vi "Read TCP FIFO MTi.vi"(6 "Error In":errorcluster, 9 "Vessel.lvclass":refnum<class "Vessel.lvclass">) -> (0 "Error Out":errorcluster, 3 "Vessel.lvclass 2":refnum<class "Vessel.lvclass">)   [LabVIEW 2014, in "Vessel.lvclass"]
uses:
  Vessel.lvclass
panel:
  out "MT_DATA":sgl[](array[numeric])
  out "MT_BITS":u8[](array[numeric])
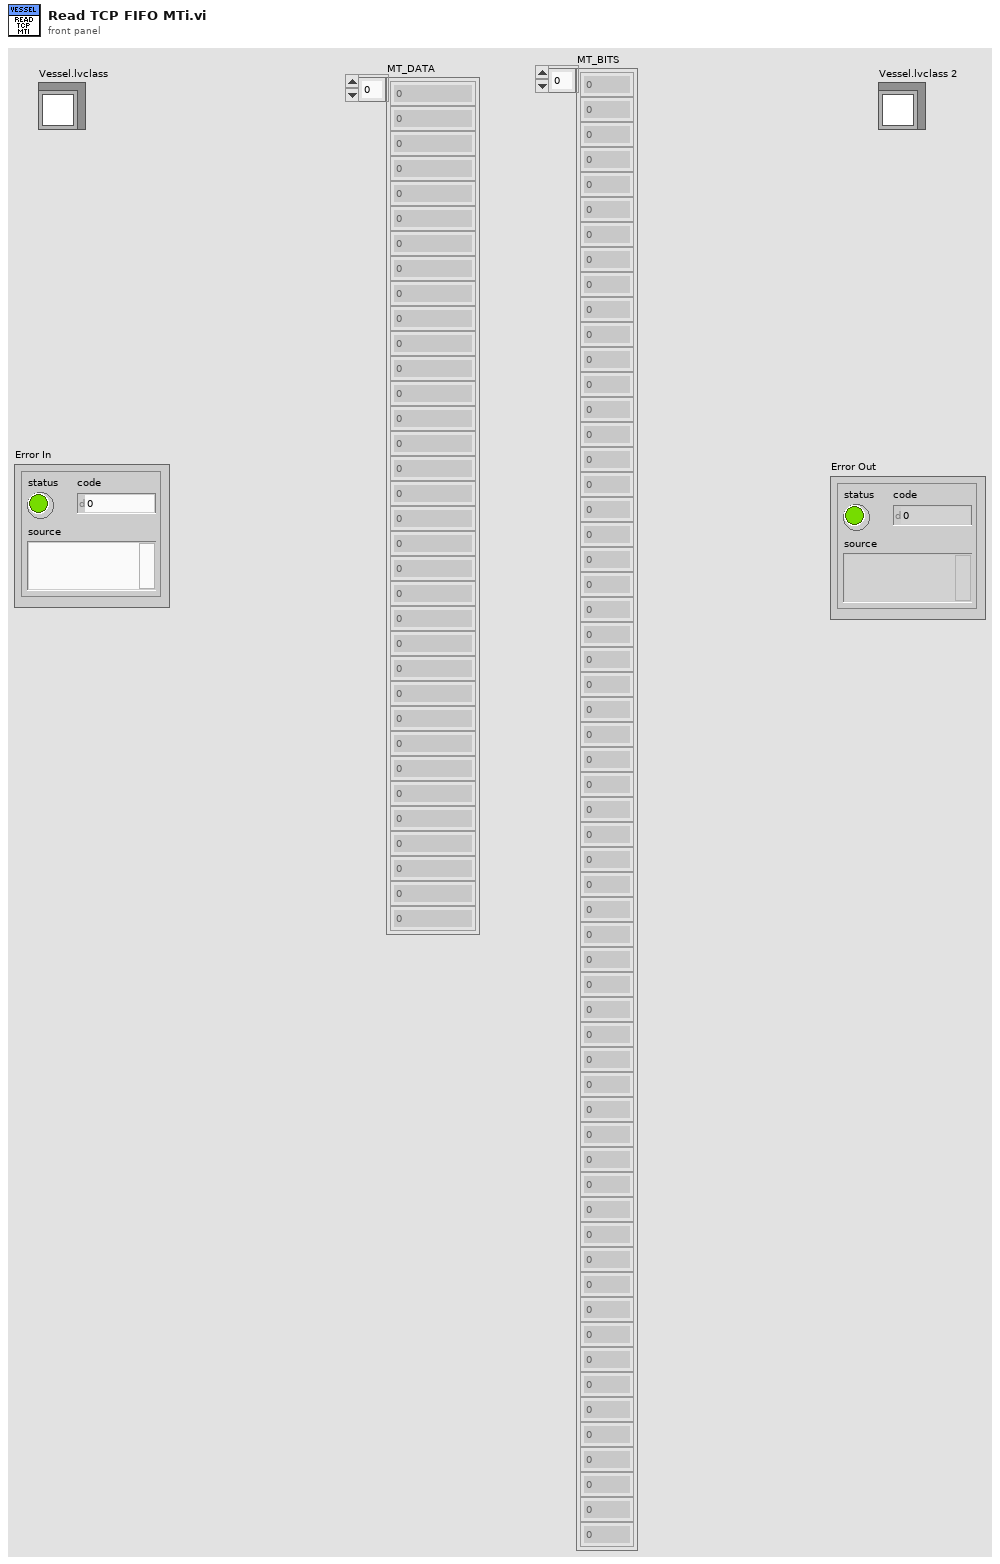
[diagram p1: front panel]
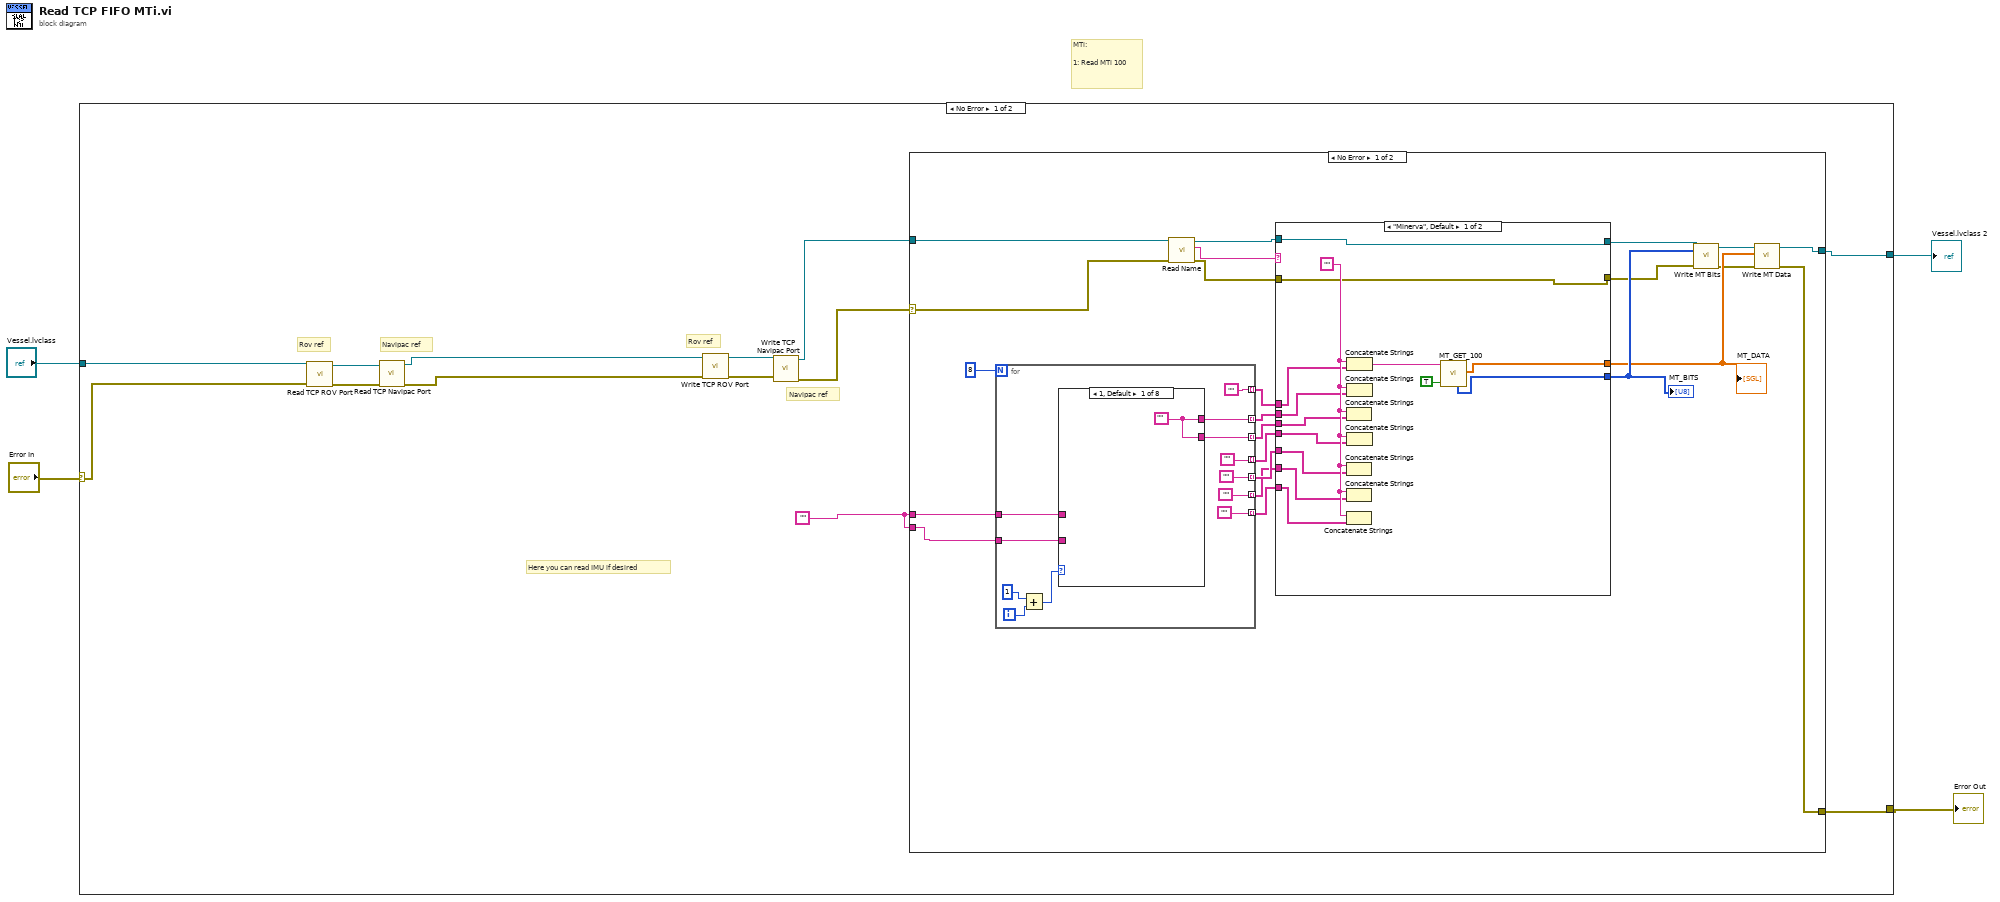
[diagram p0: block diagram]
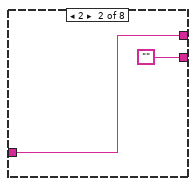
[diagram p2: hidden frame]
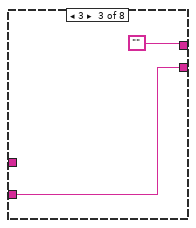
[diagram p3: hidden frame]
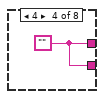
[diagram p4: hidden frame]
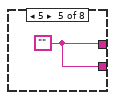
[diagram p5: hidden frame]
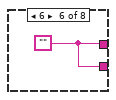
[diagram p6: hidden frame]
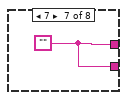
[diagram p7: hidden frame]
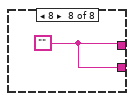
[diagram p8: hidden frame]
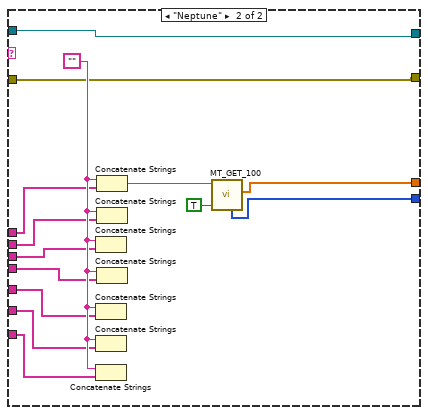
[diagram p9: hidden frame]
diagram:
  # "MTi:\n\n1: Read MTi 100"
  n1 = case shown="No Error" "Error In" {
    selector: "Error In" -> [w15 w93]
    tunnel: "Vessel.lvclass" -> [w14 w94]
    tunnel: [w17 w93] -> w2
    tunnel: [w16 w94] -> w1
    frame No Error {
      w5 = ""
      # "Here you can read IMU if desired"
      # "Navipac ref"
      # "Rov ref"
      # "Navipac ref"
      # "Rov ref"
      n2 = call-dynamic "Read TCP ROV Port.vi"("error in (no error)"=w15, "Vessel in"=w14) -> ("error out"=w12:errorcluster, "Vessel out"=w13:refnum<class "Vessel.lvclass">)  [unwired: 7 in, 1 out]
      n3 = call-dynamic "Read TCP Navipac Port.vi"("error in (no error)"=w12, "Vessel in"=w13) -> ("error out"=w6:errorcluster, "Vessel out"=w9:refnum<class "Vessel.lvclass">)  [unwired: 7 in, 1 out]
      n4 = call-dynamic "Write TCP ROV Port.vi"("error in (no error)"=w6, "Vessel in"=w9) -> ("error out"=w11:errorcluster, "Vessel out"=w8:refnum<class "Vessel.lvclass">)  [unwired: 8 in]
      n5 = call-dynamic "Write TCP Navipac Port.vi"("error in (no error)"=w11, "Vessel in"=w8) -> ("error out"=w10:errorcluster, "Vessel out"=w7:refnum<class "Vessel.lvclass">)  [unwired: 8 in]
      n6 = case shown="No Error" w10 {
        selector: w10 -> [w30 w92]
        tunnel: [w31 w92] -> w17
        tunnel: w7 -> [w38 w91]
        tunnel: [w34 w91] -> w16
        tunnel: w5 -> [w19 _]
        tunnel: w5 -> [w18 _]
        frame No Error {
          n7 = for {
            N: 8 -> [_]
            tunnel: [""] -> w23 mode=indexing
            tunnel: [""] -> w22 mode=indexing
            tunnel: [""] -> w21 mode=indexing
            tunnel: [""] -> w20 mode=indexing
            tunnel: [""] -> w26 mode=indexing
            tunnel: w19 -> [w47]
            tunnel: w18 -> [w46]
            tunnel: [w42] -> w25 mode=indexing
            tunnel: [w41] -> w24 mode=indexing
            i -> [w44]
            n8 = Add(x=1, y=w44) -> (x+y=w43:i32)
            n9 = case shown="1, Default" w43 {
              tunnel: w47 -> [_ w55 _ _ _ _ _ _]
              tunnel: w46 -> [_ _ w57 _ _ _ _ _]
              tunnel: [w53 w55 "" w58 w59 w60 w61 w62] -> w42
              tunnel: [w53 "" w57 w58 w59 w60 w61 w62] -> w41
              frame 1, Default {
                w53 = ""
              }
              frame 2 {
              }
              frame 3 {
              }
              frame 4 {
                w58 = ""
              }
              frame 5 {
                w59 = ""
              }
              frame 6 {
                w60 = ""
              }
              frame 7 {
                w61 = ""
              }
              frame 8 {
                w62 = ""
              }
            }
          }
          n10 = call-dynamic "Read Name.vi"("error in (no error)"=w30, "Vessel in"=w38) -> ("error out"=w29:errorcluster, "Name"=w39:string, "Vessel out"=w40:refnum<class "Vessel.lvclass">)  [unwired: 7 in]
          n11 = case shown="\"Minerva\", Default" w39 {
            tunnel: w23 -> [w72 w86]
            tunnel: w25 -> [w74 w88]
            tunnel: w26 -> [w75 w89]
            tunnel: w22 -> [w71 w85]
            tunnel: w24 -> [w73 w87]
            tunnel: w21 -> [w70 w84]
            tunnel: w40 -> [w67 w81]
            tunnel: w20 -> [w69 w83]
            tunnel: [w67 w81] -> w37
            tunnel: [w66 w80] -> w36
            tunnel: [w65 w79] -> w33
            tunnel: w29 -> [w63 w77]
            tunnel: [w63 w77] -> w28
            frame "Minerva", Default {
              w76 = ""
              n12 = Concatenate Strings(w76, w73) -> ()  [unwired: 1 out]
              n13 = Concatenate Strings(w76, w71) -> ()  [unwired: 1 out]
              n14 = Concatenate Strings(w76, w70) -> ()  [unwired: 1 out]
              n15 = Concatenate Strings(w76, w69) -> ()  [unwired: 1 out]
              n16 = Concatenate Strings(w76, w75) -> (w64:string)
              n17 = Concatenate Strings(w76, w74) -> ()  [unwired: 1 out]
              n18 = Concatenate Strings(w76, w72) -> ()  [unwired: 1 out]
              n19 = call "MT_GET_100.vi"("Use checksum"=TRUE, "read buffer"=w64) -> ("MT_DATA"=w65:sgl[], "MT_BITS"=w66:u8[])  [unwired: 6 in, 2 out]
            }
            frame "Neptune" {
              w90 = ""
              n20 = Concatenate Strings(w90, w87) -> ()  [unwired: 1 out]
              n21 = Concatenate Strings(w90, w85) -> ()  [unwired: 1 out]
              n22 = Concatenate Strings(w90, w84) -> ()  [unwired: 1 out]
              n23 = Concatenate Strings(w90, w83) -> ()  [unwired: 1 out]
              n24 = Concatenate Strings(w90, w89) -> (w78:string)
              n25 = Concatenate Strings(w90, w88) -> ()  [unwired: 1 out]
              n26 = Concatenate Strings(w90, w86) -> ()  [unwired: 1 out]
              n27 = call "MT_GET_100.vi"("Use checksum"=TRUE, "read buffer"=w78) -> ("MT_DATA"=w79:sgl[], "MT_BITS"=w80:u8[])  [unwired: 6 in, 2 out]
            }
          }
          "MT_BITS" <- w36
          "MT_DATA" <- w33
          n28 = call-dynamic "Write MT Bits.vi"("error in (no error)"=w28, "MT Bits"=w36, "Vessel in"=w37) -> ("error out"=w32:errorcluster, "Vessel out"=w35:refnum<class "Vessel.lvclass">)  [unwired: 7 in]
          n29 = call-dynamic "Write MT Data.vi"("error in (no error)"=w32, "MT Data"=w33, "Vessel in"=w35) -> ("error out"=w31:errorcluster, "Vessel out"=w34:refnum<class "Vessel.lvclass">)  [unwired: 7 in]
        }
        frame Error {
        }
      }
    }
    frame Error {
    }
  }
  "Vessel.lvclass 2" <- w1
  "Error Out" <- w2
